vi "VDH-reportStatus.vi"(8 "error in (no error)":errorcluster, 10 "message":string, 11 "VDH-VNA_data_handler in":refnum<class "VDH-VNA_data_handler.lvclass">) -> (0 "error out":errorcluster, 3 "VDH-VNA_data_handler out":refnum<class "VDH-VNA_data_handler.lvclass">)   [LabVIEW 2020, in "VDH-VNA_data_handler.lvlib" / "VDH-VNA_data_handler.lvclass"]
uses:
  VDH-VNA_data_handler.lvclass
  C:/Program Files (x86)/National Instruments/LabVIEW 2020/vi.lib/ActorFramework/Actor/Actor.lvclass
  common/interface/CI-common_interface/CI-status_clust.ctl
  common/interface/CI-common_interface/CI-module_enum.ctl
  <vilib>/ActorFramework/Actor/Actor.lvclass/Actor.ctl
  common/interface/CI-common_interface Messages/CI-recieveStatus Msg/CI-recieveStatus Msg.lvclass/CI-recieveStatus Msg.ctl
  <vilib>/ActorFramework/Message Enqueuer/Message Enqueuer.lvclass/Message Enqueuer.ctl
  <vilib>/ActorFramework/Message Enqueuer/Enqueue.vi
  common/interface/CI-common_interface Messages/CI-recieveStatus Msg/CI-recieveStatus Msg.lvclass
  C:/Program Files (x86)/National Instruments/LabVIEW 2020/vi.lib/ActorFramework/Message/Message.lvclass
  <vilib>/ActorFramework/Message Priority Queue/Priority Enqueue.vi
  common/interface/CI-common_interface/CI-common_interface.lvclass
  <vilib>/ActorFramework/Actor/Actor.lvclass
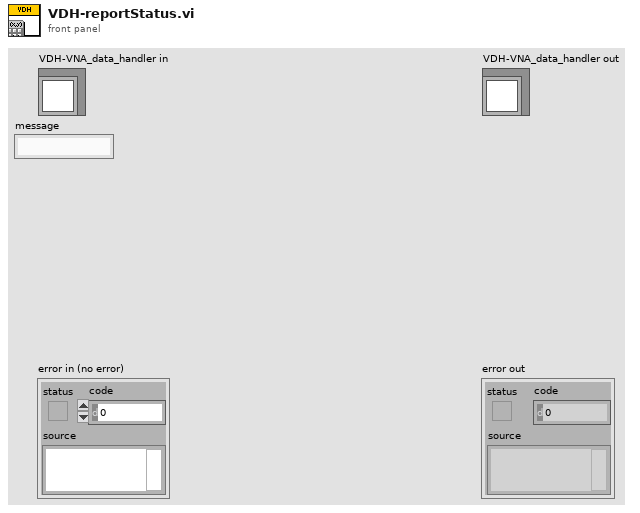
[diagram p1: front panel]
types:
  T1 = typedef "CI-common_interface.lvlib/CI-common_interface.lvclass/CI-status_clust.ctl" = cluster{"sender":T2, "message":string}
  T2 = typedef "CI-common_interface.lvlib/CI-common_interface.lvclass/CI-module_enum.ctl" = enum16{"Undefined", "HWM", "VDH", "GUI"}
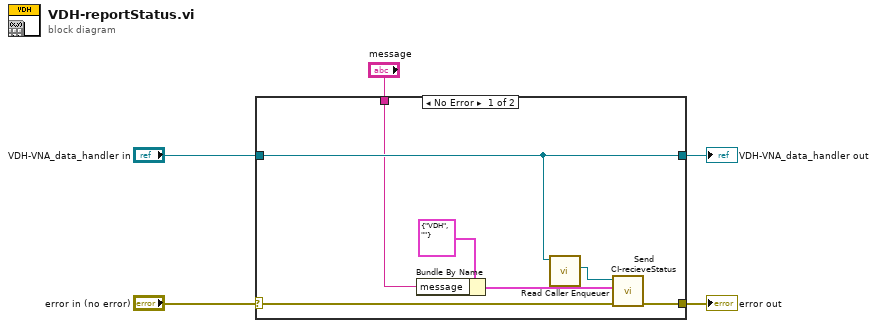
[diagram p0: block diagram]
diagram:
  n1 = case shown="No Error" "error in (no error)" {
    selector: "error in (no error)" -> [w9 w14]
    tunnel: [w8 w14] -> w4
    tunnel: [w7 w13] -> w2
    tunnel: "VDH-VNA_data_handler in" -> [w7 w13]
    tunnel: "message" -> [w6 _]
    frame No Error {
      n2 = Bundle By Name(cluster=T1 {"sender"=enum."VDH", "message"=""} ("status"), "message"=w6) -> (w10:T1)
      n3 = call <vilib>:"Read Caller Enqueuer.vi"("Actor"=w7) -> ("Caller Enqueuer"=w12:refnum<class "Message Enqueuer.lvclass">)  [unwired: 10 in]
      n4 = call "Send CI-recieveStatus.vi"("error in (no error)"=w9, "status"=w10, "Message Enqueuer"=w12) -> ("error out"=w8:errorcluster)  [unwired: 7 in, 1 out]
    }
    frame Error {
    }
  }
  "error out" <- w4
  "VDH-VNA_data_handler out" <- w2
